vi "Plot.vi"(8 "error in (no error)":errorcluster, 11 "Spectrum Recorder in":refnum<class "Spectrum Recorder.lvclass">) -> (0 "error out":errorcluster, 3 "Spectrum Recorder out":refnum<class "Spectrum Recorder.lvclass">)   [LabVIEW 2016, in "Spectrum Recorder.lvclass"]
uses:
  Spectrum Recorder.lvclass
  Spectrum Recorder.lvclass/Spectrum Recorder.ctl
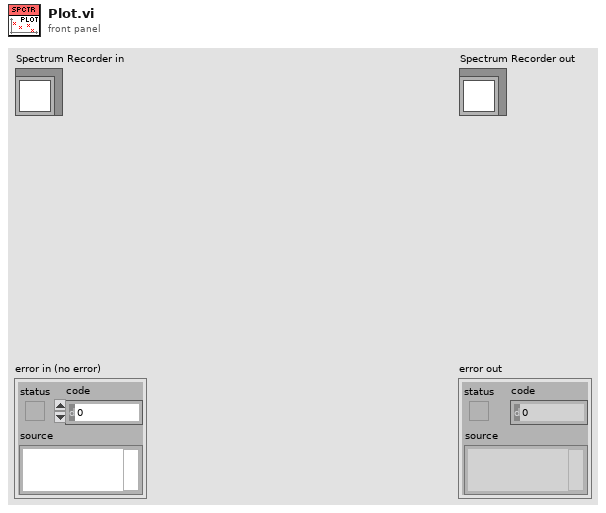
[diagram p1: front panel]
types:
  T1 = enum16{"open", "open or create", "create or replace", "create", "open (read-only)"}
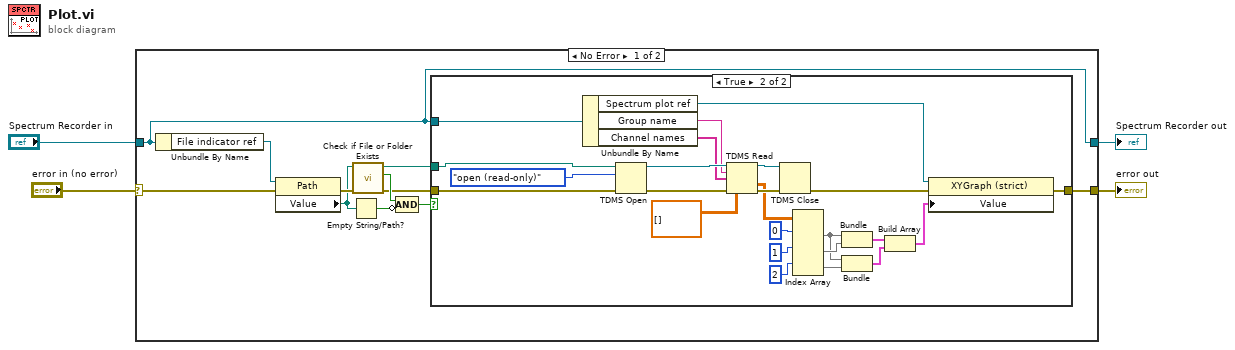
[diagram p0: block diagram]
diagram:
  n1 = case shown="No Error" "error in (no error)" {
    selector: "error in (no error)" -> [w6 w42]
    tunnel: [w5 w42] -> w3
    tunnel: [w7 w41] -> w1
    tunnel: "Spectrum Recorder in" -> [w7 w41]
    frame No Error {
      n2 = Unbundle By Name(w7) -> ("File indicator ref"=w15:refnum<vi>)
      n3 = property class="Path"(reference=w15, error in=w6) -> (error out=w14:errorcluster, "Value"=w13:path)  [unwired: 1 out]
      n4 = Empty String/Path?(string/path=w13) -> (empty?=w11:bool)
      n5 = call <vilib>:"Check if File or Folder Exists.vi"("error in (no error)"=w14, "path"=w13) -> ("error out"=w8:errorcluster, "file or folder exists?"=w12:bool, "dup path"=w9:path)  [unwired: 7 in]
      n6 = Compound Arithmetic op=AND(w12, invert w11) -> (w10:bool)
      n7 = case shown="True" w10 {
        tunnel: w9 -> [_ w36]
        tunnel: w8 -> [w16 w35]
        tunnel: w7 -> [_ w33]
        tunnel: [w16 w28] -> w5
        frame False {
        }
        frame True {
          n8 = Unbundle By Name(w33) -> ("Spectrum plot ref"=w27:refnum<vi>, "Group name"=w32:string, "Channel names"=w31:string[])
          n9 = TDMS Open(8:w35, 10:T1."open (read-only)" ("operation (0:open)"), 11:w36) -> (0:w37:errorcluster, 3:w38:refnum<k34>)  [unwired: 4 in]
          n10 = TDMS Read(0:w38, 5:w32, 7:w31, 11:w37, 12:dbl[][] []) -> (4:w39:refnum<k34>, 10:w26:dbl[][], 15:w40:errorcluster)  [unwired: 3 in, 3 out]
          n11 = TDMS Close(8:w40, 11:w39) -> (0:w29:errorcluster)  [unwired: 1 out]
          n12 = Index Array(array=w26, index (row) #1=0 ("index (row)"), index (row) #2=1 ("index (row)"), index (row) #3=2 ("index (row)")) -> (element #1=w21:dbl[], element #2=w22:dbl[], element #3=w20:dbl[])  [unwired: 3 in]
          n13 = Bundle(w21, w22) -> (w19:cluster{dbl[], dbl[]})  [unwired: 1 in]
          n14 = Bundle(w21, w20) -> (w18:cluster{dbl[], dbl[]})  [unwired: 1 in]
          n15 = Build Array(w19, w18) -> (w17:cluster{dbl[], dbl[]}[])
          n16 = property class="XYGraph (strict)"(reference=w27, error in=w29, "Value"=w17) -> (error out=w28:errorcluster)  [unwired: 1 out]
        }
      }
    }
    frame Error {
    }
  }
  "error out" <- w3
  "Spectrum Recorder out" <- w1
